vi "util.file.template.vi"(8 "error in (no error)":errorcluster, 9 "Enum":enum16{"Read", "Write"}(ring)=enum."Write", 10 "sensor_flow":T1[](array[typedef]), 11 "file path (dialog if empty)":path) -> (0 "error out":errorcluster, 2 "Array":T1[](array[typedef]), 3 "new file path (Not A Path if cancelled)":path)   [LabVIEW 2024]
uses:
  controls/UiStepBuilder.ctl
  controls/type.step-builder.ctl
  <vilib>/Utility/file.llb/Read Delimited Spreadsheet (string).vi
  <vilib>/Utility/file.llb/Write Delimited Spreadsheet (string).vi
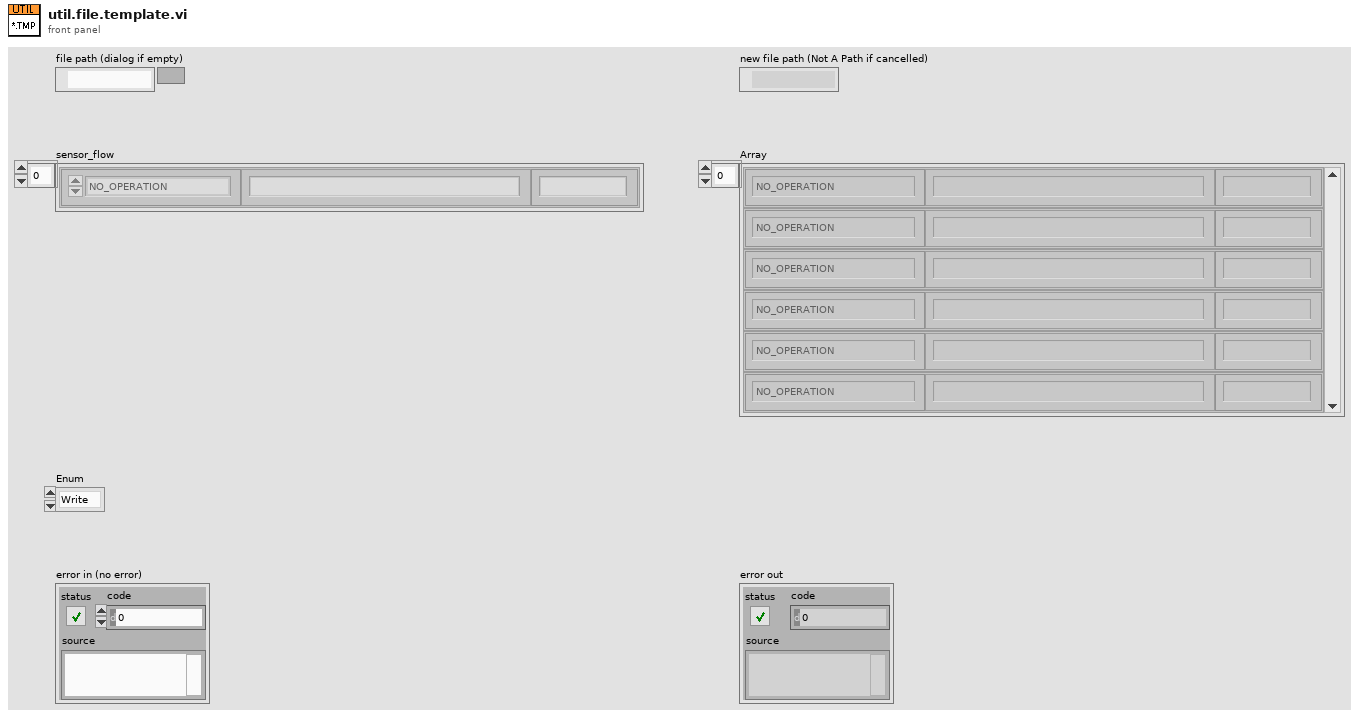
[diagram p1: front panel]
types:
  T1 = typedef "UiStepBuilder.ctl" = cluster{"Step Function":T2, "ParamString":string, "Step Label":string}
  T2 = typedef "type.step-builder.ctl" = enum16{"NO_OPERATION", "DELAY-JUMP", "DELAY", "JUMP", "COMPLETE", "SCHEDULER", "IRR-CHECK", "UNIT-CHECK", "UNIT-SAMPLE", "UNIT-DOSE", "LOG-REPORT", "LOG-MESSAGE", "IO-READ", "IO-READ-MANY", "IO-WRITE", "IO-COMPARE-OUT", "IO-COMPARE-IN", "PROC-START", "PROC-STOP", "PROC-LOAD", "PROC-IS-COMPLETED", "RECORD-MOVE", "GET-RH", "GET-UV", "GET-WD", "GET-WS", "OCS-CHECK", "OCS-RECORD"}
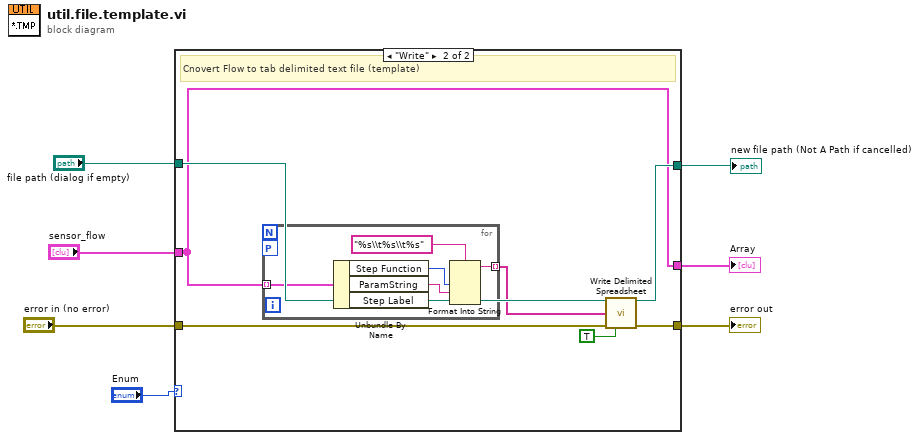
[diagram p0: block diagram]
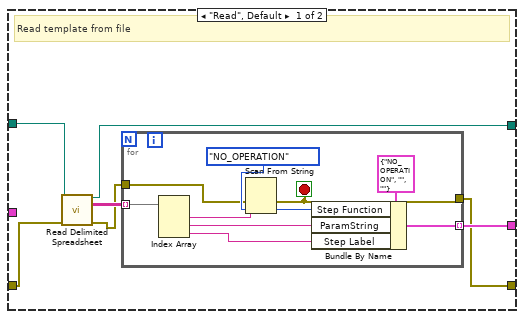
[diagram p2: hidden frame]
diagram:
  n1 = case shown="\"Write\"" "Enum" {
    tunnel: "error in (no error)" -> [w10 w31]
    tunnel: [w8 w30] -> w6
    tunnel: "sensor_flow" -> [_ w25]
    tunnel: [w11 w29] -> w4
    tunnel: "file path (dialog if empty)" -> [w13 w27]
    tunnel: [w12 w25] -> w1
    frame "Read", Default {
      # "Read template from file"
      n2 = call-poly <vilib>:"Read Delimited Spreadsheet.vi"("file path (dialog if empty)"=w13, "error in (no error)"=w10) -> ("new file path (Not A Path if cancelled)"=w11:path, "all rows"=w14:string[][], "error out"=w9:errorcluster)  [unwired: 8 in, 3 out]
      n3 = for {
        tunnel: w14 -> [w22] mode=indexing
        tunnel: [w17] -> w12 mode=indexing
        tunnel: w9 -> [w16]
        tunnel: [w15] -> w8
        stop <- w15 stop-if-true
        n4 = Index Array(array=w22) -> (element #1=w21:string, element #2=w19:string, element #3=w18:string)  [unwired: 3 in]
        n5 = Scan From String(input string=w21, error in=w16, default 1=type.step-builder."NO_OPERATION" ("UiStepFunction")) -> (error out=w15:errorcluster, output 1=w20:T2)  [unwired: 2 in, 2 out]
        n6 = Bundle By Name(cluster=T1 {"Step Function"=enum."NO_OPERATION", "ParamString"="", "Step Label"=""} ("UiBuilderStep"), "Step Function"=w20, "ParamString"=w19, "Step Label"=w18) -> (w17:T1)
      }
    }
    frame "Write" {
      # "Cnovert Flow to tab delimited text file (template)"
      n7 = for {
        tunnel: w25 -> [w36] mode=indexing
        tunnel: [w32] -> w26 mode=indexing
        workers-P: _ -> [_]
        n8 = Unbundle By Name(w36) -> ("Step Function"=w35:T2, "ParamString"=w34:string, "Step Label"=w33:string)
        n9 = Format Into String(format string="%s\\t%s\\t%s", w35, w34, w33) -> (resulting string=w32:string)  [unwired: 2 in, 1 out]
      }
      n10 = call-poly <vilib>:"Write Delimited Spreadsheet.vi"("file path (dialog if empty)"=w27, "1D data"=w26, "error in (no error)"=w31, "transpose? (no:F)"=TRUE) -> ("new file path (Not A Path if cancelled)"=w29:path, "error out"=w30:errorcluster)  [unwired: 10 in]
    }
  }
  "error out" <- w6
  "new file path (Not A Path if cancelled)" <- w4
  "Array" <- w1
